vi "publish -- eventful.vi"(7 "publisher action":T1, 10 "stepper pos IN":dbl=1000.0 format="%#_10f") -> (0 "request":refnum<user-event>, 1 "response":refnum<user-event>, 2 "stepper pos OUT":dbl=1000.0 format="%#_10f")   [LabVIEW 2018]
uses:
  publisher action.ctl
  publisher message.ctl
  publisher message -- request.ctl
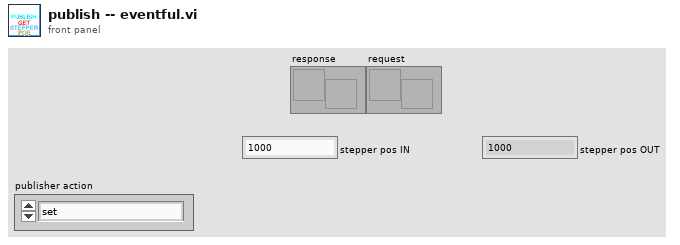
[diagram p1: front panel]
types:
  T1 = typedef "publisher action.ctl" = enum16{"set", "get", "init", "--send request", "--wait", "--respond", "init writer", "init reader"}
  T2 = typedef "publisher message -- request.ctl" = cluster{"message action":enum16{"next?", "ok"}}
  T3 = typedef "publisher message.ctl" = cluster{"action":enum16{"next?", "ok"}, "data":dbl}
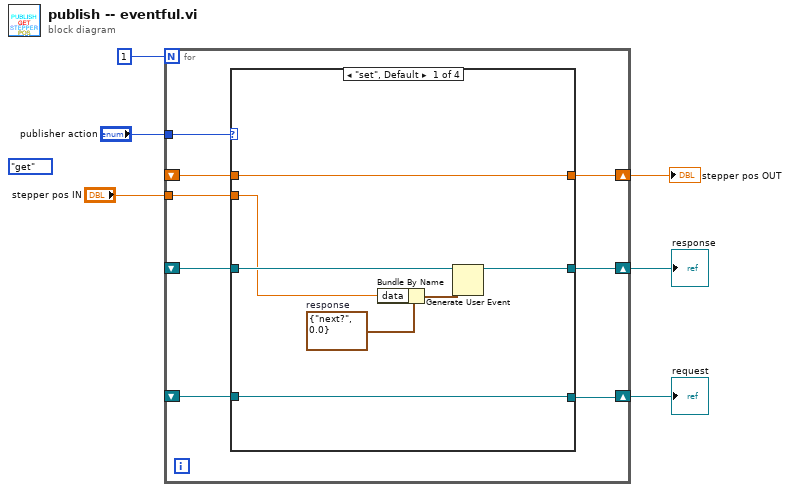
[diagram p0: block diagram]
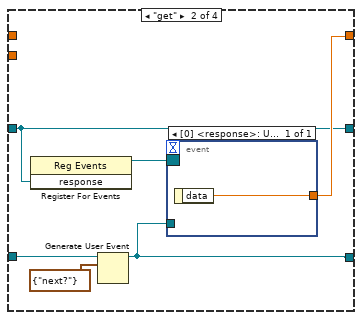
[diagram p2: hidden frame]
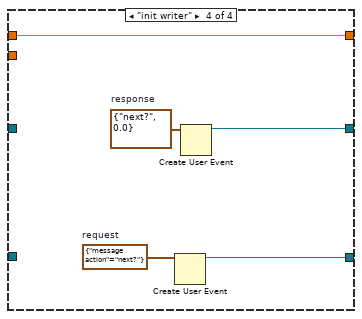
[diagram p4: hidden frame]
diagram:
  (unwired) publisher_action."get" ("publisher action")
  n1 = for {
    N: 1 -> [_]
    tunnel: "publisher action" -> [w14]
    tunnel: "stepper pos IN" -> [w12]
    shift-right: [w13] -> w3
    shift-left: _ -> [w11]
    shift-right: [w7] -> w2
    shift-left: _ -> [w10]
    shift-right: [w8] -> w1
    shift-left: _ -> [w9]
    n2 = case shown="\"set\", Default" w14 {
      tunnel: [w21 w26 w29 w32] -> w13
      tunnel: w12 -> [w15 _ _ _]
      tunnel: w11 -> [w21 _ w29 w32]
      tunnel: w10 -> [w20 w25 w31 _]
      tunnel: w9 -> [w18 w24 w30 _]
      tunnel: [w18 w22 w30 w33] -> w8
      tunnel: [w19 w25 w31 w34] -> w7
      frame "set", Default {
        w16 = T3 {"action"=enum."next?", "data"=0.0}  # response
        n3 = Bundle By Name(cluster=w16, "data"=w15) -> (w17:T3)
        n4 = Generate User Event(user event=w20, event data cluster=w17) -> (user event out=w19:refnum<user-event>)  [unwired: 2 in, 1 out]
      }
      frame "get" {
        n5 = register-events(w25) -> (reference out=w27:refnum<event-registration>)  [unwired: 2 in, 1 out]
        n6 = Generate User Event(user event=w24, event data cluster=T2 {"message action"=enum."next?"} ("event data")) -> (user event out=w22:refnum<user-event>)  [unwired: 2 in, 1 out]
        n7 = event shown="[0] <response>: User Event" {
          selector: w27 -> [_]
          dyn-events: _ -> [_]
          timeout: _ -> [_]
          tunnel: [w28] -> w26
          tunnel: w22 -> [_]
          event User Event {
            n8 = event-data() -> ("data"=w28:dbl)  [unwired: 1 in]
          }
        }
      }
      frame "init reader" {
      }
      frame "init writer" {
        w35 = T2 {"message action"=enum."next?"}  # request
        w36 = T3 {"action"=enum."next?", "data"=0.0}  # response
        n9 = Create User Event(user event datatype=w35) -> (user event=w33:refnum<user-event>)  [unwired: 1 in, 1 out]
        n10 = Create User Event(user event datatype=w36) -> (user event=w34:refnum<user-event>)  [unwired: 1 in, 1 out]
      }
    }
  }
  "stepper pos OUT" <- w3
  "response" <- w2
  "request" <- w1
